vi "SaveState.vi"(3 "tabs":refnum<vi>, 4 "camera":string, 5 "file":path) -> ()   [LabVIEW 2010]
uses:
  <vilib>/addons/h5labview/H5F_mode.ctl
  <vilib>/addons/h5labview/H5File.lvlib
  <vilib>/addons/h5labview/H5GroupObject.lvlib
  <vilib>/addons/h5labview/H5Attrib.lvlib
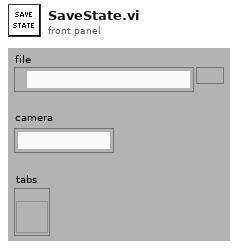
[diagram p1: front panel]
types:
  T1 = typedef "H5File.lvlib/H5F_mode.ctl" = enum16{"read-only", "read-write", "overwrite", "create new", "open or create"}
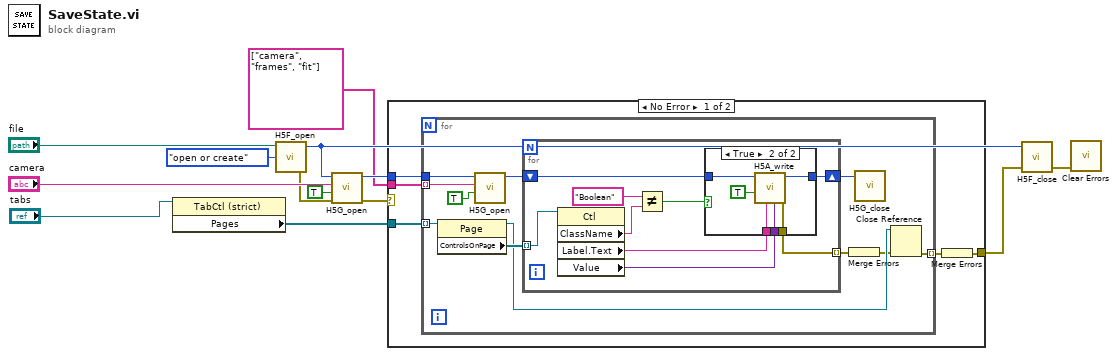
[diagram p0: block diagram]
diagram:
  n1 = property class="TabCtl (strict)"(reference="tabs") -> ("Pages"=w1:refnum<vi>[])  [unwired: 1 in, 2 out]
  n2 = call <vilib>:"H5F_open.vi"("mode"=H5F_mode."open or create", "path"="file") -> ("error out"=w8:errorcluster, "ref"=w9:i32)  [unwired: 2 in]
  n3 = call <vilib>:"H5G_open.vi"("error in (no error)"=w8, "create? (F)"=TRUE, "name"="camera", "ref"=w9) -> ("error out"=w7:errorcluster, "group"=w6:i32)  [unwired: 2 in]
  n4 = case shown="No Error" w7 {
    tunnel: w6 -> [w18 _]
    tunnel: string[] ["camera", "frames", "fit"] -> [w17 _]
    tunnel: [w15 _] -> w4
    tunnel: w1 -> [w14 _]
    frame No Error {
      n5 = for {
        tunnel: w18 -> [w29]
        tunnel: w17 -> [w28] mode=indexing
        tunnel: [w27] -> w16 mode=indexing
        tunnel: w14 -> [w19] mode=indexing
        n6 = property class="Page"(reference=w19) -> (reference out=w25:refnum<vi>, "ControlsOnPage"=w26:refnum<vi>[])  [unwired: 1 in, 1 out]
        n7 = call <vilib>:"H5G_open.vi"("create? (F)"=TRUE, "name"=w28, "ref"=w29) -> ("group"=w23:i32)  [unwired: 3 in, 1 out]
        n8 = for {
          tunnel: w26 -> [w38] mode=indexing
          shift-right: [w35] -> w21
          shift-left: w23 -> [w37]
          tunnel: [w34] -> w24 mode=indexing
          n9 = property class="Ctl"(reference=w38) -> ("ClassName"=w31:string, "Label.Text"=w36:string, "Value"=w33:variant)  [unwired: 1 in, 2 out]
          n10 = Not Equal?(x="Boolean" ("Class Name"), y=w31) -> (x != y?=w30:bool)
          n11 = case shown="True" w30 {
            tunnel: w37 -> [w39 w45]
            tunnel: w36 -> [_ w44]
            tunnel: [w39 w43] -> w35
            tunnel: [_ w42] -> w34
            tunnel: w33 -> [_ w41]
            frame False {
            }
            frame True {
              n12 = call <vilib>:"H5A_write.vi"("value"=w41, "attrib_name"=w44, "overwrite? (F)"=TRUE, "ref"=w45) -> ("error out"=w42:errorcluster, "ref out"=w43:i32)  [unwired: 4 in]
            }
          }
        }
        n13 = Merge Errors(w24) -> (w20:errorcluster)
        n14 = call <vilib>:"H5G_close.vi"("ref"=w21) -> ()  [unwired: 4 in, 1 out]
        n15 = Close Reference(reference=w25, error in (no error)=w20) -> (error out=w27:errorcluster)
      }
      n16 = Merge Errors(w16) -> (w15:errorcluster)
    }
    frame Error {
    }
  }
  n17 = call <vilib>:"H5F_close.vi"("error in (no error)"=w4, "ref"=w9) -> ("error out"=w2:errorcluster)  [unwired: 3 in]
  n18 = call <vilib>:"Clear Errors.vi"("error in (no error)"=w2) -> ()  [unwired: 6 in, 1 out]
